vi "autonomous mode.vi"() -> ()   [LabVIEW 2012, in "Robot Green.lvrbt"]
uses:
  Robot Green.lvrbt
  <vilib>/NXT/Hardware/Plugins/Tetrix DC Motor/TetrixDCMotorAddress.ctl
  <vilib>/NXT/NXTIO Xnodes/NXTIONodeSubVIs/TETRIX IO Check Battery.vi
  <vilib>/NXT/Dual Mode Library/Waits/Wait_Num(msec).vi
  <vilib>/NXT/NXTIO Xnodes/NXTIONodeSubVIs/TETRIX IO Stop DC Motors.vi
  <vilib>/NXT/Dual Mode Library/Waits/Wait_Num.vi
  <vilib>/NXT/NXTIO Xnodes/NXTIONodeSubVIs/TETRIX IO Move DC Motors.vi
  <vilib>/NXT/Subs/LVHSConnector.ctl
  <vilib>/NXT/NXTIO Xnodes/AddressXNode/NXTIOAddress.xnode
  <vilib>/NXT/NXTIO Xnodes/NXTIOXNode/NXTIO.xnode
  <vilib>/NXT/LegoClasses/BrickReference/BrickReference.lvclass
panel:
  out "Enabled":bool
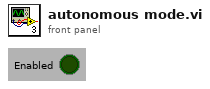
[diagram p1: front panel]
types:
  T1 = typedef "TetrixDCMotorAddress.ctl" = i32
  T2 = typedef "LVHSConnector.ctl" = refnum<class "BrickReference.lvclass">
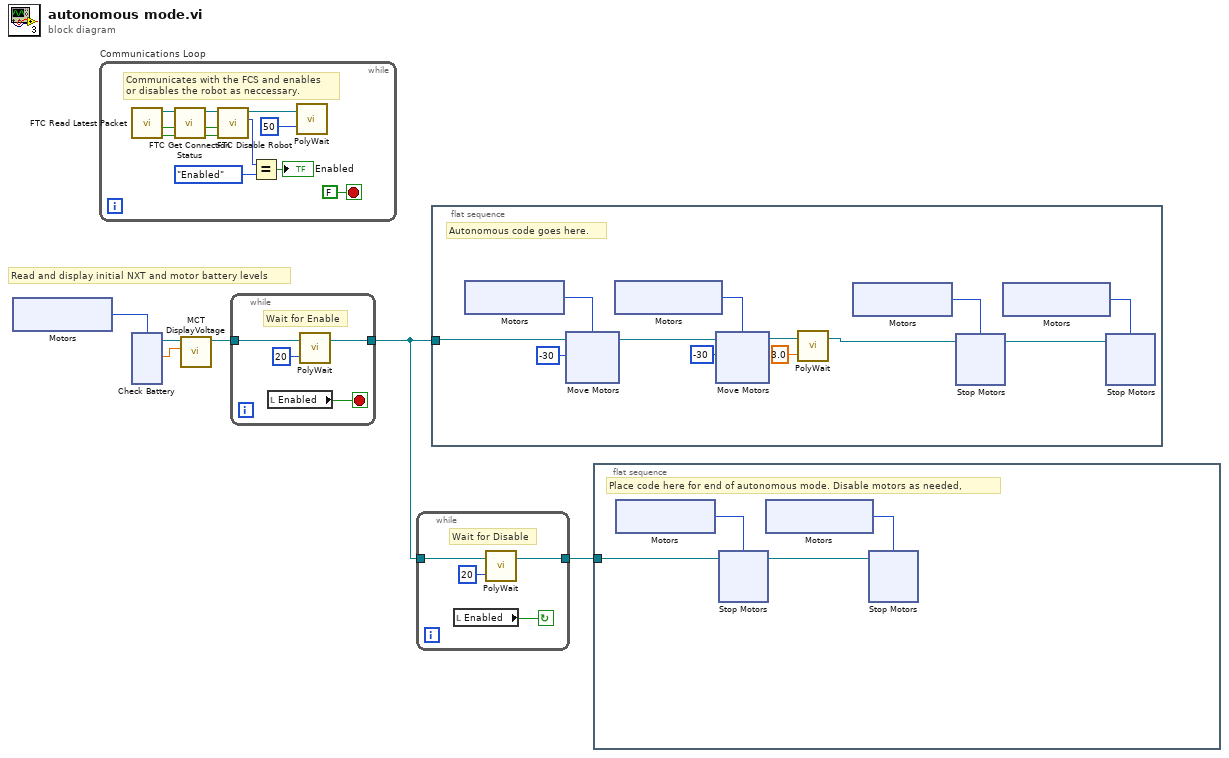
[diagram p0: block diagram]
diagram:
  # "Read and display initial NXT and motor battery levels"
  n1 = xnode "Motors"() -> ("Motor"=w6:T1)
  n2 = while "Communications Loop" {
    stop <- FALSE stop-if-true
    # "Communicates with the FCS and enables \nor disables the robot as neccessary."
    n3 = call <vilib>:"FTC Read Latest Packet.vi"() -> ("Packet Received?"=w16:bool, "Stopped?"=w15:bool, "NXT/EV3"=w18:T2)  [unwired: 6 in, 3 out]
    n4 = call <vilib>:"FTC Get Connection Status.vi"("Packet Received?"=w16, "Stopped?"=w15, "NXT/EV3"=w18) -> ("Online?"=w7:bool, "Stopped?"=w8:bool, "NXT/EV3"=w17:T2)  [unwired: 5 in]
    n5 = call <vilib>:"FTC Disable Robot.vi"("Online?"=w7, "Stopped?"=w8, "NXT/EV3"=w17) -> ("Enabled?"=w11:enum16{"Disabled", "Enabled"}, "NXT/EV3"=w13:T2)  [unwired: 3 in]
    n6 = Equal?(x=w11, y=enum16{"Disabled", "Enabled"}."Enabled") -> (x = y?=→"Enabled":bool)
    n7 = call-poly <vilib>:"PolyWait.vi"("Time (100 msec)"=u32 50 ("Time (msec)"), "NXT/EV3"=w13) -> ()  [unwired: 2 in, 1 out]
  }
  n8 = xnode "Check Battery"("Motors"=w6) -> ("Voltage 1"=w1:sgl, "NXT/EV3"=w3:T2)  [unwired: 1 in]
  n9 = call <vilib>:"MCT DisplayVoltage.vi"("Motor Voltage"=w1, "NXT/EV3"=w3) -> ("NXT/EV3"=w2:T2)  [unwired: 9 in]
  n10 = while {
    tunnel: [w20] -> w5
    tunnel: w2 -> [w19]
    stop <- w21 stop-if-true
    # "Wait for Enable"
    n11 = local read "Enabled"() -> (w21:bool)
    n12 = call-poly <vilib>:"PolyWait.vi"("Time (100 msec)"=u32 20 ("Time (msec)"), "NXT/EV3"=w19) -> ("NXT/EV3"=w20:T2)  [unwired: 2 in]
  }
  n13 = while {
    tunnel: [w24] -> w4
    tunnel: w5 -> [w23]
    stop <- w25 continue-if-true
    # "Wait for Disable"
    n14 = local read "Enabled"() -> (w25:bool)
    n15 = call-poly <vilib>:"PolyWait.vi"("Time (100 msec)"=u32 20 ("Time (msec)"), "NXT/EV3"=w23) -> ("NXT/EV3"=w24:T2)  [unwired: 2 in]
  }
  n16 = flat-sequence {
    tunnel: w5 -> [w35]
    frame #0 {
      # "Autonomous code goes here."
      n17 = xnode "Motors"() -> ("Motor"=w36:T1)
      n18 = xnode "Move Motors"("Power/Speed 1"=i8 -30, "Motors"=w36, "NXT/EV3"=w35) -> ("NXT/EV3"=w38:T2)
      n19 = xnode "Motors"() -> ("Motor"=w37:T1)
      n20 = xnode "Move Motors"("Power/Speed 1"=i8 -30, "Motors"=w37, "NXT/EV3"=w38) -> ("NXT/EV3"=w32:T2)
      n21 = call-poly <vilib>:"PolyWait.vi"("Time (1 sec)"=sgl 3.0, "NXT/EV3"=w32) -> ("NXT/EV3"=w27:T2)  [unwired: 2 in]
      n22 = xnode "Motors"() -> ("Motor"=w28:T1)
      n23 = xnode "Stop Motors"("Motors"=w28, "NXT/EV3"=w27) -> ("NXT/EV3"=w30:T2)
      n24 = xnode "Motors"() -> ("Motor"=w29:T1)
      n25 = xnode "Stop Motors"("Motors"=w29, "NXT/EV3"=w30) -> ()  [unwired: 1 out]
    }
  }
  n26 = flat-sequence {
    tunnel: w4 -> [w70]
    frame #0 {
      # "Place code here for end of autonomous mode. Disable motors as needed,"
      n27 = xnode "Motors"() -> ("Motor"=w69:T1)
      n28 = xnode "Stop Motors"("Motors"=w69, "NXT/EV3"=w70) -> ("NXT/EV3"=w67:T2)
      n29 = xnode "Motors"() -> ("Motor"=w68:T1)
      n30 = xnode "Stop Motors"("Motors"=w68, "NXT/EV3"=w67) -> ()  [unwired: 1 out]
    }
  }
